vi "Build Unregister Status Message.vi"(0 "CSM Name":string, 5 "Source CSM Name (* as Default)":string="*", 7 "Status":string) -> (6 "State with Arguments":string)   [LabVIEW 2020, in "Communicable State Machine.lvlib"]
doc: "Builds unregister status message. The message looks like:\n[source-state]@[source-module] >> [response-module] -><unregister>\nFor examples:\nDownloadFinished@Downloader >> StartPlay -><unregister>\nDownloadFinished@Downloader -><unregister>\n\n<b>Inputs:</b>\n - <b>Source CSM Name (* as Default)</b>:\n - <b>CSM Name</b>:\n - <b>Status</b>:\n\n<b>Outputs:</b>\n - <b>State with Arguments</b>:"
uses:
  Communicable State Machine.lvlib
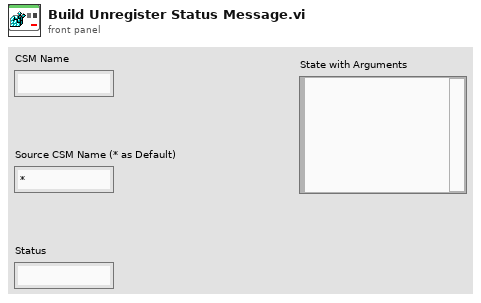
[diagram p1: front panel]
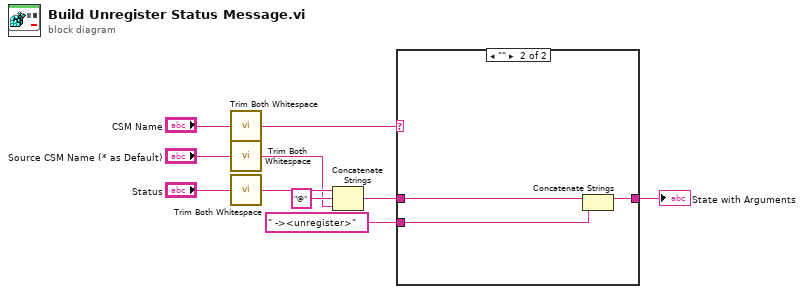
[diagram p0: block diagram]
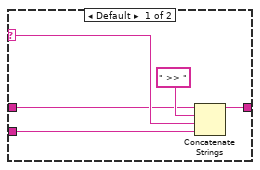
[diagram p2: hidden frame]
diagram:
  n1 = call "Trim Both Whitespace.vi"("string"="CSM Name") -> ("trimmed string"=w3:string)  [unwired: 1 in]
  n2 = call "Trim Both Whitespace.vi"("string"="Source CSM Name (* as Default)") -> ("trimmed string"=w4:string)  [unwired: 1 in]
  n3 = call "Trim Both Whitespace.vi"("string"="Status") -> ("trimmed string"=w6:string)  [unwired: 1 in]
  n4 = Concatenate Strings(w6, "@" ("string"), w4) -> (w2:string)
  n5 = case shown="\"\"" w3 {
    selector: w3 -> [w14 _]
    tunnel: [w15 w18] -> w10
    tunnel: w2 -> [w12 w17]
    tunnel: " -><unregister>" ("string") -> [w11 w16]
    frame Default {
      n6 = Concatenate Strings(w12, " >> " ("string"), w14, w11) -> (w15:string)
    }
    frame "" {
      n7 = Concatenate Strings(w17, w16) -> (w18:string)
    }
  }
  "State with Arguments" <- w10
